vi "Sine_wave R4.vi"() -> (3 "waveform":sgl[][](array[numeric]))   [LabVIEW 2018]
uses:
  <vilib>/measure/NI_MABase.lvlib
panel:
  in  "meas. time":dbl
  in  "dt FPGA":dbl
  in  "sampling info":cluster{"Fs":dbl, "#s":dbl}={"Fs"=1000.0, "#s"=1000.0} {"Fs" format="%.2p"}
  in  "amplitude\n[V]":dbl
  in  "Frequency \n[1/s]":dbl
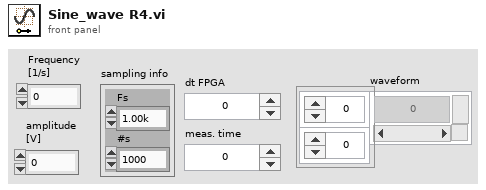
[diagram p1: front panel]
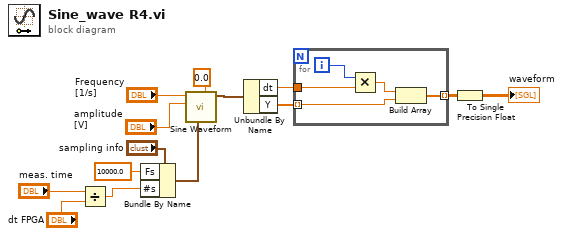
[diagram p0: block diagram]
diagram:
  n1 = Divide(x="meas. time", y="dt FPGA") -> (x/y=w5:dbl)
  n2 = Bundle By Name(cluster="sampling info", "Fs"=10000.0, "#s"=w5) -> (w3:cluster{"Fs":dbl, "#s":dbl})
  n3 = call <vilib>:"Sine Waveform.vi"("offset"=0.0, "sampling info"=w3, "amplitude"="amplitude\n[V]", "frequency"="Frequency \n[1/s]") -> ("signal out"=w14:waveform(dbl))  [unwired: 6 in, 1 out]
  n4 = Unbundle By Name(w14) -> ("dt"=w9:dbl, "Y"=w10:dbl[])
  n5 = for {
    tunnel: w10 -> [w19] mode=indexing
    tunnel: w9 -> [w17]
    tunnel: [w15] -> w2 mode=indexing
    i -> [w18]
    n6 = Multiply(x=w18, y=w17) -> (x*y=w16:dbl)
    n7 = Build Array(w16, w19) -> (w15:dbl[])
  }
  n8 = To Single Precision Float(number=w2) -> (single precision float=→"waveform":sgl[][])
